vi "DAQ_change_405.vi"(2 "error in":errorcluster, 3 "405":dbl) -> (0 "error out":errorcluster)   [LabVIEW 2015]
uses:
  GLOBAL/Global_DAQ.vi
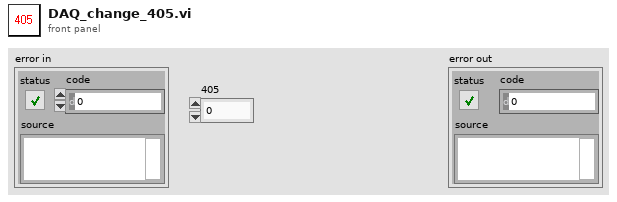
[diagram p1: front panel]
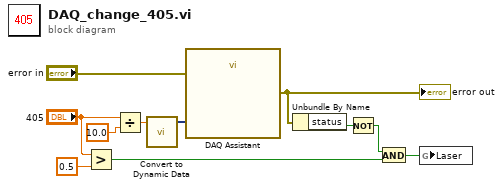
[diagram p0: block diagram]
diagram:
  n1 = Greater?(x="405", y=0.5) -> (0:w7:bool)
  n2 = Divide(x="405", y=10.0) -> (x/y=w10:dbl)
  n3 = call "Convert to Dynamic Data"("Double"=w10) -> ("Dynamic Data Type"=w11:dynamicdata)  [unwired: 3 in]
  n4 = call "DAQ Assistant"("data"=w11, "error in"="error in") -> ("error out"=w3:errorcluster)  [unwired: 16 in, 1 out]
  "error out" <- w3
  n5 = Unbundle By Name(w3) -> ("status"=w9:bool)
  n6 = Not(x=w9) -> (.not. x?=w8:bool)
  n7 = And(x=w8, y=w7) -> (x .and. y?=w1:bool)
  n8 = global write "Global_DAQ.vi" "Laser"(w1) -> ()
